vi "KE622x -- Get Trig Output Line.vi"(0 "Resource In":refnum<visa-resource-name>, 1 "Check For SCPI Errors? (T)":bool=TRUE, 11 "error in (no error)":errorcluster) -> (4 "Resource Out (dupl)":refnum<visa-resource-name>, 8 "Trig Output Line":T1, 15 "error out":errorcluster)   [LabVIEW 2019, in "Keithley 622x.lvlib"]
uses:
  Keithley 622x.lvlib
  Typedefs/KE622x -- Trig Link Line.ctl
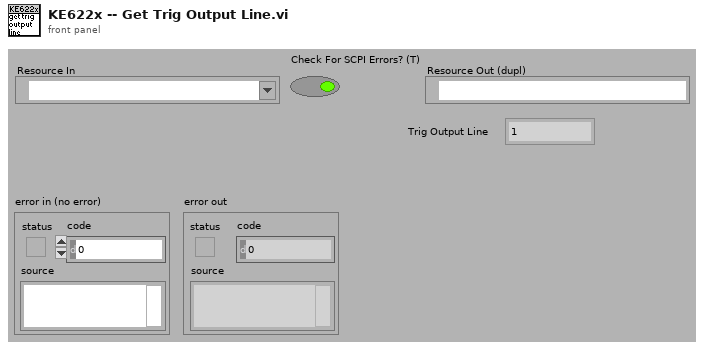
[diagram p1: front panel]
types:
  T1 = typedef "Keithley 622x.lvlib/KE622x -- Trig Link Line.ctl" = enum16{"1", "2", "3", "4", "5", "6"}
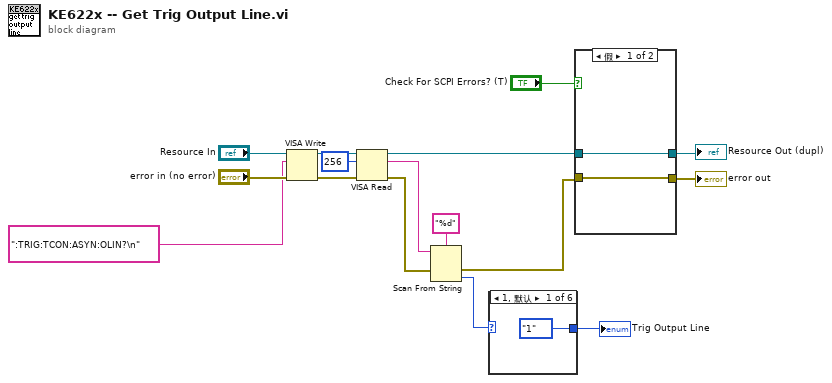
[diagram p0: block diagram]
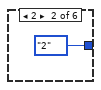
[diagram p2: hidden frame]
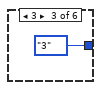
[diagram p3: hidden frame]
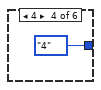
[diagram p4: hidden frame]
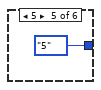
[diagram p5: hidden frame]
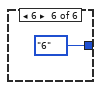
[diagram p6: hidden frame]
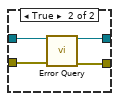
[diagram p7: hidden frame]
diagram:
  n1 = VISA Write(VISA resource name="Resource In", write buffer=":TRIG:TCON:ASYN:OLIN?\n" ("format string"), error in (no error)="error in (no error)") -> (VISA resource name out=w10:refnum<visa-resource-name>, error out=w9:errorcluster)  [unwired: 1 out]
  n2 = VISA Read(VISA resource name=w10, byte count=u32 256, error in (no error)=w9) -> (VISA resource name out=w3:refnum<visa-resource-name>, read buffer=w5:string, error out=w7:errorcluster)  [unwired: 1 out]
  n3 = Scan From String(format string="%d", input string=w5, error in=w7) -> (error out=w4:errorcluster, output 1=w2:i32)  [unwired: 2 in, 2 out]
  n4 = case shown="1, 默认" w2 {
    tunnel: [KE622x_--_Trig_Link_Line."1" ("Arm Extern Input Line") KE622x_--_Trig_Link_Line."2" ("Arm Extern Input Line") KE622x_--_Trig_Link_Line."3" ("Arm Extern Input Line") KE622x_--_Trig_Link_Line."4" ("Arm Extern Input Line") KE622x_--_Trig_Link_Line."5" ("Arm Extern Input Line") KE622x_--_Trig_Link_Line."6" ("Arm Extern Input Line")] -> w1
    frame 1, Default {
    }
    frame 2 {
    }
    frame 3 {
    }
    frame 4 {
    }
    frame 5 {
    }
    frame 6 {
    }
  }
  "Trig Output Line" <- w1
  n5 = case shown="假" "Check For SCPI Errors? (T)" {
    tunnel: w3 -> [w24 w28]
    tunnel: w4 -> [w23 w27]
    tunnel: [w23 w26] -> w12
    tunnel: [w24 w25] -> w13
    frame False {
    }
    frame True {
      n6 = call "Error Query.vi"("VISA Resource In"=w28, "error in (no error)"=w27) -> ("VISA Resource Out (dupl)"=w25:refnum<visa-resource-name>, "error out"=w26:errorcluster)  [unwired: 10 in, 2 out]
    }
  }
  "Resource Out (dupl)" <- w13
  "error out" <- w12
